vi "Teleop.vi"(10 "Match Info":T1={"Autonomous Elapsed Seconds"=0.0, "TeleOp Elapsed Seconds"=0.0, "Disabled Elapsed Seconds"=0.0, "Visited Autonomous"=FALSE, "Visited TeleOp"=FALSE, "Visited Disabled"=FALSE, "Autonomous Settings"={"Autonomous Style"=enum."Independent", "VI Refnum"=refnum}}, 11 "Call Context":T2) -> ()   [LabVIEW 2012]
doc: "This VI is called for each TeleOp packet received from the DS where the robot is not disabled. It is often used to read from the joysticks and update I/O or to update setpoints for timed control loops. It should complete and return within 20 milliseconds or it may miss DS packets."
uses:
  <vilib>/Rock Robotics/WPI/DriverStation/WPI_DriverStationDerivedRobotMode.ctl
  <vilib>/Rock Robotics/WPI/DriverStation/WPI_DriverStationMatch Info.ctl
  <vilib>/Rock Robotics/WPI/Relay/WPI_RelayValue.ctl
  Robot Global Data.vi
  <vilib>/Rock Robotics/WPI/Joystick/WPI_JoystickGetSetRefNum.vi
panel:
  in  "Dep Const":dbl=0.5
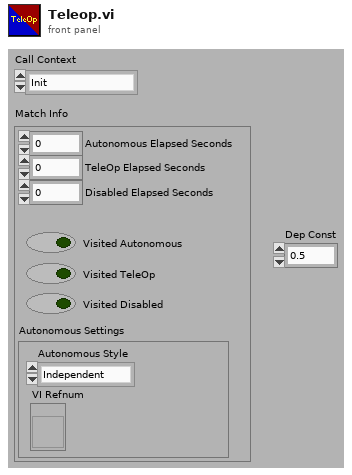
[diagram p1: front panel]
types:
  T1 = typedef "WPI_DriverStationMatch Info.ctl" = cluster{"Autonomous Elapsed Seconds":dbl, "TeleOp Elapsed Seconds":dbl, "Disabled Elapsed Seconds":dbl, "Visited Autonomous":bool, "Visited TeleOp":bool, "Visited Disabled":bool, "Autonomous Settings":cluster{"Autonomous Style":enum16{"Iterative", "Independent"}, "VI Refnum":refnum<vi>}}
  T2 = typedef "WPI_DriverStationDerivedRobotMode.ctl" = enum16{"Init", "Execute", "Stop"}
  T3 = typedef "WPI_RelayValue.ctl" = enum16{"Off", "On", "Forward", "Reverse"}
  T4 = typedef "WPI_ServoDeviceRef.ctl" = cluster{"DeviceStatus":errorcluster, "Digital Module":T5, "PWM Channel":T6, "DeadBand":T7}
  T5 = typedef "FPGA_TypedefDigitalModule.ctl" = enum16{"Digital Module 1", "Digital Module 2"}
  T6 = typedef "FPGA_DIOPWMChannel.ctl" = enum8{"PWM 1", "PWM 2", "PWM 3", "PWM 4", "PWM 5", "PWM 6", "PWM 7", "PWM 8", "PWM 9", "PWM 10", "Invalid"}
  T7 = typedef "WPI_PWMDeadband.ctl" = cluster{"Name":string, "maxPositivePwm":i32, "minPositivePwm":i32, "centerPwm":i32, "maxNegativePwm":i32, "minNegativePwm":i32, "angularRange":u16}
  T8 = typedef "WPI_MotorControlDeviceRef.ctl" = cluster{"DeviceStatus":errorcluster, "Type":enum16{"PWM", "CAN"}, "PWM":cluster{"Digital Module":T5, "PWM Channel":T6, "DeadBand":T7}, "CAN":cluster{"Device Number":u8, "Control Mode":T9, "Semaphore":T10, "Max Vout":dbl}, "Invert":bool, "TransformRef":T11, "InvTransformRef":T11}
  T9 = typedef "WPI_CANJaguar_ControlMode.ctl" = enum8{"Percent VBus", "Current", "Speed", "Position", "Voltage"}
  T10 = typedef "Semaphore RefNum" = refnum<k1>
  T11 = typedef "WPI_PWMTransform_ConPane.ctl" = refnum<vi>
  T12 = cluster{"Driver Station Digital Input (1-8)[0]":bool, "Driver Station Digital Input (1-8)[1]":bool, "Driver Station Digital Input (1-8)[2]":bool, "Driver Station Digital Input (1-8)[3]":bool, "Driver Station Digital Input (1-8)[4]":bool, "Driver Station Digital Input (1-8)[5]":bool, "Driver Station Digital Input (1-8)[6]":bool, "Driver Station Digital Input (1-8)[7]":bool, "Driver Station Digital Input (1-8)[8]":bool}
  T13 = cluster{"Right Servo High":dbl, "Right Servo Mid":dbl, "Right Servo Low":dbl, "Left Servo High":dbl, "Left Servo Mid":dbl, "Left Servo Low":dbl}
  T14 = typedef "WPI_JoystickDevRef.ctl" = cluster{"Device":T15}
  T15 = typedef "WPI_JoystickDeviceEnum.ctl" = enum16{"USB 1", "USB 2", "USB 3", "USB 4", "Kinect 1", "Kinect 2"}
  T16 = cluster{"axis 1 (x)":dbl, "axis 2 (y)":dbl, "axis 3 (throttle)":dbl, "axis 4":dbl, "axis 5":dbl, "axis 6":dbl}
  T17 = typedef "WPI_JoystickButtonState.ctl" = cluster{"Button 1":bool, "Button 2":bool, "Button 3":bool, "Button 4":bool, "Button 5":bool, "Button 6":bool, "Button 7":bool, "Button 8":bool, "Button 9":bool, "Button 10":bool, "Button 11":bool, "Button 12":bool}
  T18 = typedef "WPI_RelayDevRef.ctl" = cluster{"DevStatus":errorcluster, "Relay Channel":T19, "Digital Module":T5, "Relay Direction":T20}
  T19 = typedef "FPGA_DIORelayChannel.ctl" = enum8{"Relay 1", "Relay 2", "Relay 3", "Relay 4", "Relay 5", "Relay 6", "Relay 7", "Relay 8", "Invalid"}
  T20 = typedef "WPI_RelayDirection.ctl" = enum16{"Both directions", "Forward only", "Reverse only"}
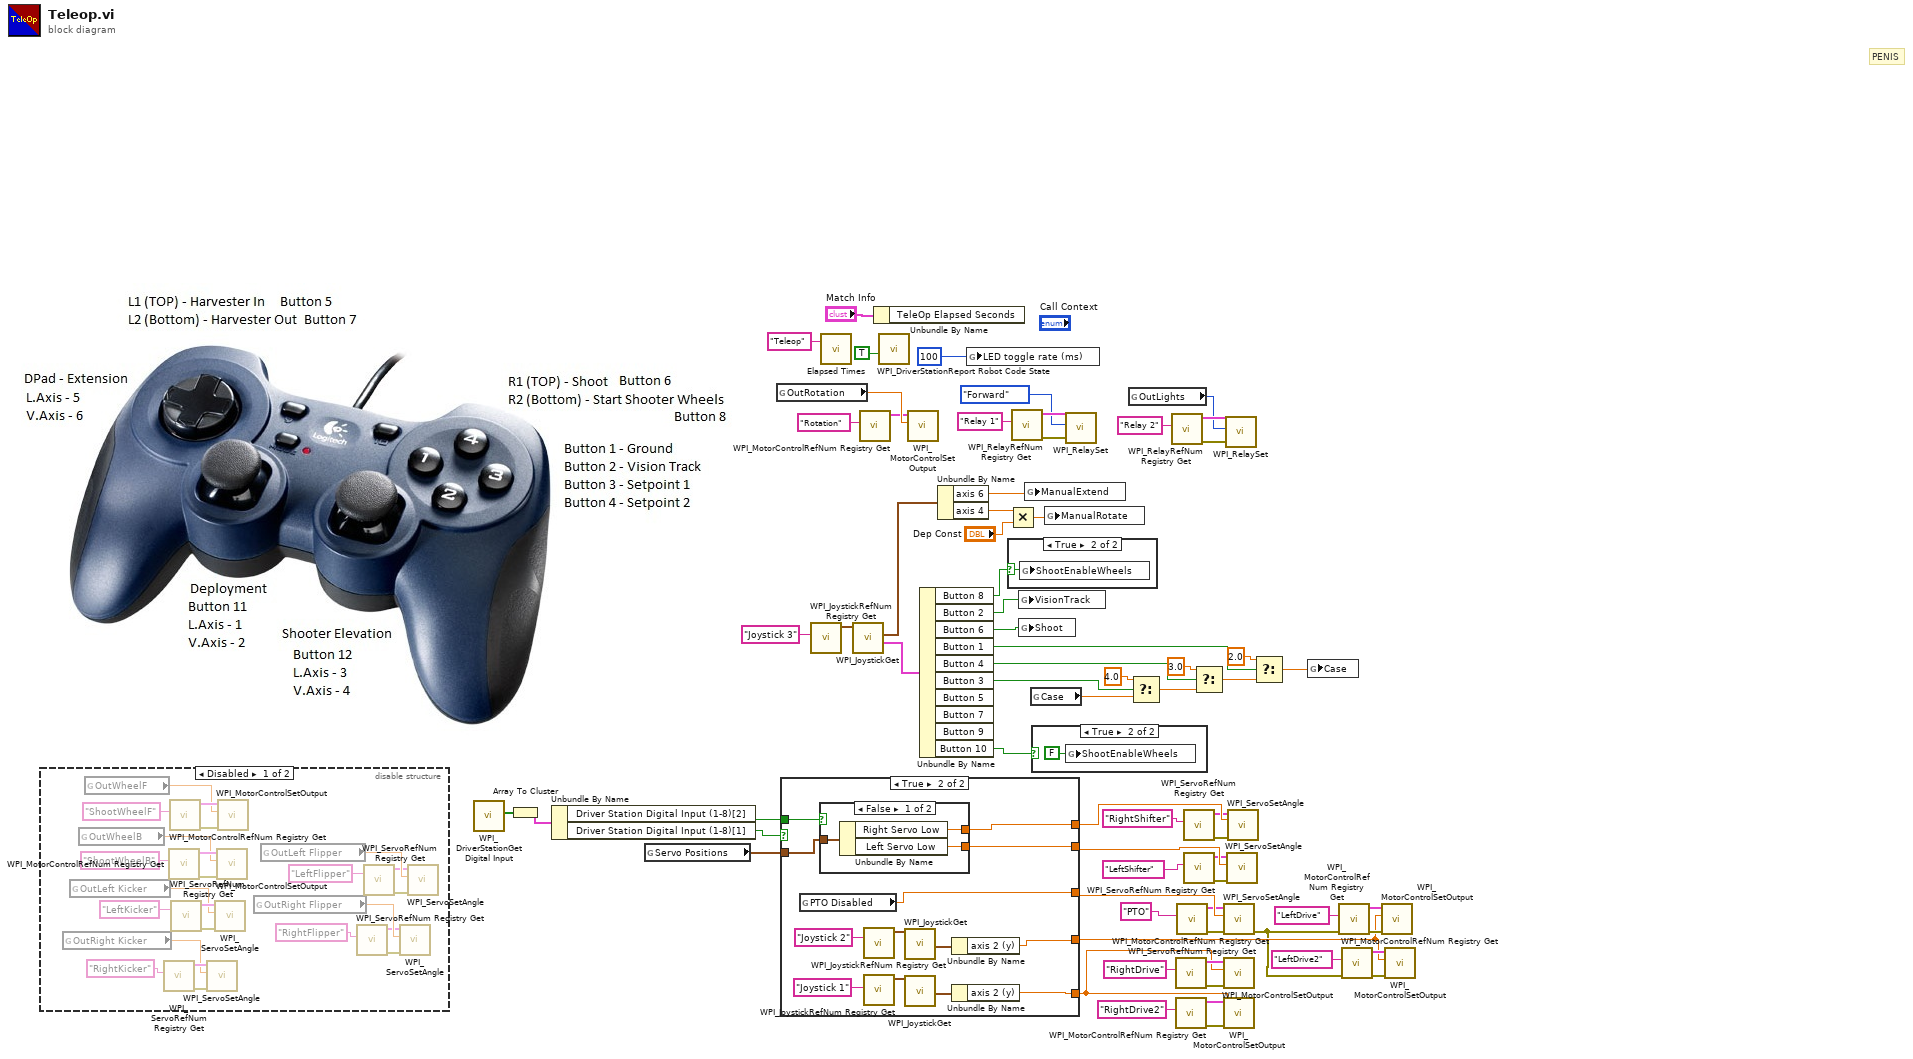
[diagram p0: block diagram]
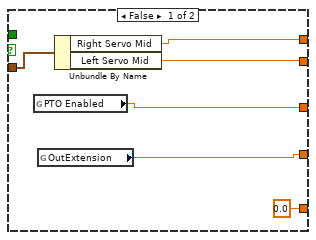
[diagram p3: hidden frame]
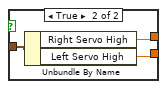
[diagram p4: hidden frame]
diagram:
  # "PENIS"
  n1 = disable-structure shown="Disabled" {
    frame Disabled {
      n2 = global read "Robot Global Data.vi" "OutRight Kicker"() -> (w78:dbl)
      n3 = global read "Robot Global Data.vi" "OutLeft Kicker"() -> (w79:dbl)
      n4 = global read "Robot Global Data.vi" "OutWheelB"() -> (w86:dbl)
      n5 = global read "Robot Global Data.vi" "OutWheelF"() -> (w87:dbl)
      n6 = call <vilib>:"WPI_ServoRefNum Registry Get.vi"("refnum name"="RightKicker") -> ("error out"=w83:errorcluster, "ServoDeviceRef"=w82:T4)  [unwired: 9 in]
      n7 = call <vilib>:"WPI_MotorControlRefNum Registry Get.vi"("refnum name"="ShootWheelB") -> ("error out"=w89:errorcluster, "MotorControlDevRef"=w90:T8)  [unwired: 9 in]
      n8 = call <vilib>:"WPI_MotorControlRefNum Registry Get.vi"("refnum name"="ShootWheelF") -> ("error out"=w91:errorcluster, "MotorControlDevRef"=w88:T8)  [unwired: 9 in]
      n9 = call <vilib>:"WPI_ServoRefNum Registry Get.vi"("refnum name"="LeftKicker") -> ("error out"=w84:errorcluster, "ServoDeviceRef"=w80:T4)  [unwired: 9 in]
      n10 = call <vilib>:"WPI_ServoSetAngle.vi"("error in (no error)"=w83, "Angle"=w78, "ServoDeviceRef"=w82) -> ()  [unwired: 7 in, 2 out]
      n11 = call <vilib>:"WPI_ServoSetAngle.vi"("error in (no error)"=w84, "Angle"=w79, "ServoDeviceRef"=w80) -> ()  [unwired: 7 in, 2 out]
      n12 = call <vilib>:"WPI_MotorControlSetOutput.vi"("error in (no error)"=w89, "Output"=w86, "MotorControlDevRef"=w90) -> ()  [unwired: 6 in, 3 out]
      n13 = call <vilib>:"WPI_MotorControlSetOutput.vi"("error in (no error)"=w91, "Output"=w87, "MotorControlDevRef"=w88) -> ()  [unwired: 6 in, 3 out]
      n14 = global read "Robot Global Data.vi" "OutRight Flipper"() -> (w77:dbl)
      n15 = global read "Robot Global Data.vi" "OutLeft Flipper"() -> (w76:dbl)
      n16 = call <vilib>:"WPI_ServoRefNum Registry Get.vi"("refnum name"="RightFlipper") -> ("error out"=w72:errorcluster, "ServoDeviceRef"=w73:T4)  [unwired: 9 in]
      n17 = call <vilib>:"WPI_ServoRefNum Registry Get.vi"("refnum name"="LeftFlipper") -> ("error out"=w71:errorcluster, "ServoDeviceRef"=w75:T4)  [unwired: 9 in]
      n18 = call <vilib>:"WPI_ServoSetAngle.vi"("error in (no error)"=w72, "Angle"=w77, "ServoDeviceRef"=w73) -> ()  [unwired: 7 in, 2 out]
      n19 = call <vilib>:"WPI_ServoSetAngle.vi"("error in (no error)"=w71, "Angle"=w76, "ServoDeviceRef"=w75) -> ()  [unwired: 7 in, 2 out]
    }
    frame Enabled {
    }
  }
  n20 = call <vilib>:"WPI_DriverStationGet Digital Input.vi"() -> ("Driver Station Digital Input (1-8)"=w35:bool[])  [unwired: 11 in]
  n21 = Array To Cluster(array=w35) -> (cluster=w34:T12)
  n22 = Unbundle By Name(w34) -> ("Driver Station Digital Input (1-8)[2]"=w33:bool, "Driver Station Digital Input (1-8)[1]"=w25:bool)
  n23 = global read "Robot Global Data.vi" "Servo Positions"() -> (w32:T13)
  n24 = global read "Robot Global Data.vi" "OutRotation"() -> (w19:dbl)
  n25 = case shown="True" w25 {
    tunnel: w33 -> [_ w112]
    tunnel: w32 -> [w99 w111]
    tunnel: [w98 w110] -> w31
    tunnel: [w97 w109] -> w30
    tunnel: [w96 w108] -> w22
    tunnel: [w94 w101] -> w21
    tunnel: [0.0 w100] -> w20
    frame False {
      n26 = global read "Robot Global Data.vi" "PTO Enabled"() -> (w96:dbl)
      n27 = global read "Robot Global Data.vi" "OutExtension"() -> (w94:dbl)
      n28 = Unbundle By Name(w99) -> ("Right Servo Mid"=w98:dbl, "Left Servo Mid"=w97:dbl)
    }
    frame True {
      n29 = global read "Robot Global Data.vi" "PTO Disabled"() -> (w108:dbl)
      n30 = case shown="False" w112 {
        tunnel: w111 -> [w115 w118]
        tunnel: [w114 w117] -> w110
        tunnel: [w113 w116] -> w109
        frame False {
          n31 = Unbundle By Name(w115) -> ("Right Servo Low"=w114:dbl, "Left Servo Low"=w113:dbl)
        }
        frame True {
          n32 = Unbundle By Name(w118) -> ("Right Servo High"=w117:dbl, "Left Servo High"=w116:dbl)
        }
      }
      n33 = call <vilib>:"WPI_JoystickRefNum Registry Get.vi"("refnum name"="Joystick 2") -> ("JoystickDevRef"=w102:T14)  [unwired: 1 in, 9 out]
      n34 = call <vilib>:"WPI_JoystickRefNum Registry Get.vi"("refnum name"="Joystick 1") -> ("JoystickDevRef"=w106:T14)  [unwired: 1 in, 9 out]
      n35 = call <vilib>:"WPI_JoystickGet.vi"("JoystickDevRef"=w102) -> ("Axes"=w104:T16)  [unwired: 1 in, 5 out]
      n36 = call <vilib>:"WPI_JoystickGet.vi"("JoystickDevRef"=w106) -> ("Axes"=w107:T16)  [unwired: 1 in, 5 out]
      n37 = Unbundle By Name(w104) -> ("axis 2 (y)"=w101:dbl)
      n38 = Unbundle By Name(w107) -> ("axis 2 (y)"=w100:dbl)
    }
  }
  n39 = call <vilib>:"WPI_JoystickRefNum Registry Get.vi"("refnum name"="Joystick 3") -> ("JoystickDevRef"=w66:T14)  [unwired: 9 in, 1 out]
  n40 = call "Elapsed Times.vi"("Call Name"="Teleop") -> ()  [unwired: 2 in, 1 out]
  n41 = call <vilib>:"WPI_JoystickGet.vi"("JoystickDevRef"=w66) -> ("Buttons"=w64:T17, "Axes"=w63:T16)  [unwired: 4 in, 1 out]
  n42 = call <vilib>:"WPI_MotorControlRefNum Registry Get.vi"("refnum name"="Rotation") -> ("MotorControlDevRef"=w17:T8)  [unwired: 9 in, 1 out]
  n43 = Unbundle By Name("Match Info") -> ()  [unwired: 1 out]
  n44 = call <vilib>:"WPI_DriverStationReport Robot Code State.vi"("TeleOp"=TRUE ("Autonomous")) -> ()  [unwired: 10 in, 1 out]
  n45 = call <vilib>:"WPI_MotorControlSetOutput.vi"("Output"=w19, "MotorControlDevRef"=w17) -> ()  [unwired: 7 in, 3 out]
  n46 = Unbundle By Name(w64) -> ("Button 8"=w50:bool, "Button 2"=w61:bool, "Button 6"=w62:bool, "Button 1"=w60:bool, "Button 4"=w58:bool, "Button 3"=w57:bool, "Button 10"=w49:bool)  [unwired: 3 out]
  n47 = Unbundle By Name(w63) -> ("axis 6"=w9:dbl, "axis 4"=w12:dbl)
  n48 = global write "Robot Global Data.vi" "LED toggle rate (ms)"(u32 100 ("LED ms toggle rate")) -> ()
  n49 = Multiply(x=w12, y="Dep Const") -> (x*y=w10:dbl)
  n50 = case shown="True" w50 {
    selector: w50 -> [_ w119]
    frame False {
    }
    frame True {
      n51 = global write "Robot Global Data.vi" "ShootEnableWheels"(w119) -> ()
    }
  }
  n52 = call <vilib>:"WPI_RelayRefNum Registry Get.vi"("refnum name"="Relay 1") -> ("error out"=w6:errorcluster, "RelayDevRef"=w8:T18)  [unwired: 9 in]
  n53 = global write "Robot Global Data.vi" "VisionTrack"(w61) -> ()
  n54 = global write "Robot Global Data.vi" "Shoot"(w62) -> ()
  n55 = global write "Robot Global Data.vi" "ManualExtend"(w9) -> ()
  n56 = global read "Robot Global Data.vi" "Case"() -> (w52:dbl)
  n57 = case shown="True" w49 {
    frame False {
    }
    frame True {
      n58 = global write "Robot Global Data.vi" "ShootEnableWheels"(FALSE ("ShootStartWheels")) -> ()
    }
  }
  n59 = global write "Robot Global Data.vi" "ManualRotate"(w10) -> ()
  n60 = call <vilib>:"WPI_RelaySet.vi"("error in (no error)"=w6, "RelayValue"=WPI_RelayValue."Forward", "RelayDevRef"=w8) -> ()  [unwired: 7 in, 2 out]
  n61 = global read "Robot Global Data.vi" "OutLights"() -> (w1:T3)
  n62 = Select(t=4.0, s=w57, f=w52) -> (s? t:f=w56:dbl)
  n63 = call <vilib>:"WPI_RelayRefNum Registry Get.vi"("refnum name"="Relay 2") -> ("error out"=w4:errorcluster, "RelayDevRef"=w2:T18)  [unwired: 9 in]
  n64 = call <vilib>:"WPI_MotorControlRefNum Registry Get.vi"("refnum name"="RightDrive") -> ("error out"=w45:errorcluster, "MotorControlDevRef"=w47:T8)  [unwired: 9 in]
  n65 = call <vilib>:"WPI_MotorControlRefNum Registry Get.vi"("refnum name"="RightDrive2") -> ("error out"=w38:errorcluster, "MotorControlDevRef"=w36:T8)  [unwired: 9 in]
  n66 = call <vilib>:"WPI_ServoRefNum Registry Get.vi"("refnum name"="PTO") -> ("error out"=w15:errorcluster, "ServoDeviceRef"=w16:T4)  [unwired: 9 in]
  n67 = call <vilib>:"WPI_ServoRefNum Registry Get.vi"("refnum name"="RightShifter") -> ("error out"=w26:errorcluster, "ServoDeviceRef"=w27:T4)  [unwired: 9 in]
  n68 = call <vilib>:"WPI_ServoRefNum Registry Get.vi"("refnum name"="LeftShifter") -> ("error out"=w28:errorcluster, "ServoDeviceRef"=w29:T4)  [unwired: 9 in]
  n69 = Select(t=3.0, s=w58, f=w56) -> (s? t:f=w54:dbl)
  n70 = call <vilib>:"WPI_ServoSetAngle.vi"("error in (no error)"=w15, "Angle"=w22, "ServoDeviceRef"=w16) -> ("error out"=w11:errorcluster)  [unwired: 7 in, 1 out]
  n71 = call <vilib>:"WPI_MotorControlSetOutput.vi"("error in (no error)"=w45, "Output"=w20, "MotorControlDevRef"=w47) -> ()  [unwired: 6 in, 3 out]
  n72 = call <vilib>:"WPI_MotorControlSetOutput.vi"("error in (no error)"=w38, "Output"=w20, "MotorControlDevRef"=w36) -> ()  [unwired: 6 in, 3 out]
  n73 = call <vilib>:"WPI_RelaySet.vi"("error in (no error)"=w4, "RelayValue"=w1, "RelayDevRef"=w2) -> ()  [unwired: 7 in, 2 out]
  n74 = call <vilib>:"WPI_ServoSetAngle.vi"("error in (no error)"=w28, "Angle"=w30, "ServoDeviceRef"=w29) -> ()  [unwired: 7 in, 2 out]
  n75 = call <vilib>:"WPI_ServoSetAngle.vi"("error in (no error)"=w26, "Angle"=w31, "ServoDeviceRef"=w27) -> ()  [unwired: 7 in, 2 out]
  n76 = Select(t=2.0, s=w60, f=w54) -> (s? t:f=w51:dbl)
  n77 = global write "Robot Global Data.vi" "Case"(w51) -> ()
  n78 = call <vilib>:"WPI_MotorControlRefNum Registry Get.vi"("error in (no error)"=w11, "refnum name"="LeftDrive") -> ("error out"=w40:errorcluster, "MotorControlDevRef"=w43:T8)  [unwired: 8 in]
  n79 = call <vilib>:"WPI_MotorControlRefNum Registry Get.vi"("error in (no error)"=w11, "refnum name"="LeftDrive2") -> ("error out"=w39:errorcluster, "MotorControlDevRef"=w41:T8)  [unwired: 8 in]
  n80 = call <vilib>:"WPI_MotorControlSetOutput.vi"("error in (no error)"=w40, "Output"=w21, "MotorControlDevRef"=w43) -> ()  [unwired: 6 in, 3 out]
  n81 = call <vilib>:"WPI_MotorControlSetOutput.vi"("error in (no error)"=w39, "Output"=w21, "MotorControlDevRef"=w41) -> ()  [unwired: 6 in, 3 out]
